vi "ATSh_BeforeAsyncRead.vi"(0 "Handle":u32, 7 "Channel":T2, 9 "RecordsPerBuffer":u32, 11 "RecordsCount":u32, 12 "ReadSamples":T1, 13 "cFlags":u32=1) -> (4 "Handle_Out":u32, 15 "Return Code":u32)   [LabVIEW 2014]
doc: "_____AlazarTech, Scope_____\n\nConfigures a board for asynchronous AutoDMA transfers from on-board to host memory\nHandle as input."
uses:
  ATS_ctl/ATS_DMA_Channel.ctl
  ATS_ctl/ATS_ReadSamples.ctl
  ATSApi.dll
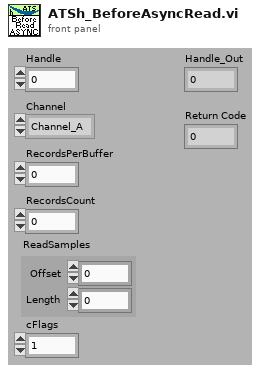
[diagram p1: front panel]
types:
  T1 = typedef "ATS_ReadSamples.ctl" = cluster{"Offset":i32, "Length":u32}
  T2 = typedef "ATS_DMA_Channel.ctl" = enum16{"Channel_A", "Channel_B", "A & B"}
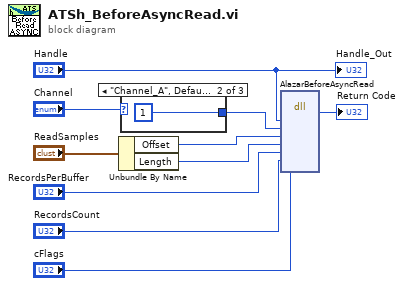
[diagram p0: block diagram]
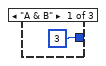
[diagram p2: hidden frame]
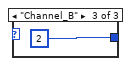
[diagram p3: hidden frame]
diagram:
  n1 = Unbundle By Name("ReadSamples") -> ("Offset"=w5:i32, "Length"=w4:u32)
  n2 = case shown="\"Channel_A\", Default" "Channel" {
    tunnel: [u32 3 ("Operation") u32 1 ("Operation") u32 2 ("Operation")] -> w6
    frame "A & B" {
    }
    frame "Channel_A", Default {
    }
    frame "Channel_B" {
    }
  }
  n3 = dll-call lib="D:/IntensityOCT/trunk/ATSApi.dll" fn="AlazarBeforeAsyncRead"("Handle"="Handle", "ChannelSelect"=w6, "TransferOffset"=w5, "TransferLength"=w4, "RecordsPerBuffer"="RecordsPerBuffer", "RecordsCount"="RecordsCount", "cFlags"="cFlags") -> (→"Return Code":u32)  [unwired: 10 in, 2 out]
  "Handle_Out" <- "Handle"
